vi "Polynomentwicklung IAG.vi"(9 "P(x)":dbl[](array[numeric]) min=0.0 max=127.0 format="%#.2f", 11 "a":dbl) -> (3 "P(a)":dbl)   [LabVIEW 2020, in "Linearisierung v2.lvlib"]
uses:
  Linearisierung v2.lvlib
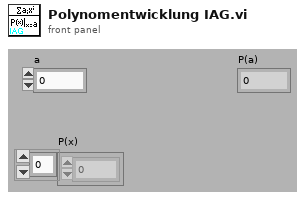
[diagram p1: front panel]
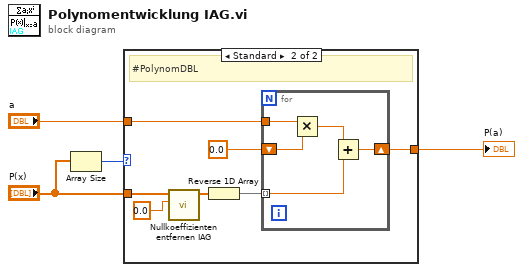
[diagram p0: block diagram]
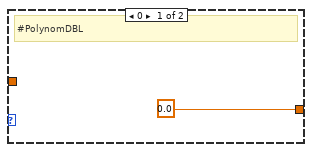
[diagram p2: hidden frame]
diagram:
  n1 = Array Size(array="P(x)") -> (size(s)=w1:i32)
  n2 = case shown="Standard" w1 {
    tunnel: "a" -> [_ w10]
    tunnel: [0.0 w9] -> w3
    tunnel: "P(x)" -> [_ w8]
    frame 0 {
      # "#PolynomDBL"
    }
    frame Default {
      # "#PolynomDBL"
      n3 = call "Nullkoeffizienten entfernen IAG.vi"("threshold"=0.0, "P(x) In"=w8) -> ("P(x) Out"=w7:dbl[])  [unwired: 8 in, 1 out]
      n4 = Reverse 1D Array(array=w7) -> (reversed array=w11:dbl[])
      n5 = for {
        shift-right: [w13] -> w9
        shift-left: 0.0 -> [w16]
        tunnel: w10 -> [w17]
        tunnel: w11 -> [w15] mode=indexing
        n6 = Multiply(x=w17, y=w16) -> (x*y=w14:dbl)
        n7 = Add(x=w14, y=w15) -> (x+y=w13:dbl)
      }
    }
  }
  "P(a)" <- w3
